vi "GSP_GT_Global.vi"() -> ()   [LabVIEW 2015]
uses:
  SystemUtil/MotorStates.ctl
  SystemUtil/ThreadStates.ctl
panel:
  in  "Grating #":i32
  in  "Grating Name":string
  in  "GT Thread state":T1
  in  "Current Grating":T2
  in  "Detent Pos":i32=6580
  in  "GT Motor State":T3
  in  "GT Position":i32
  in  "GT Target":i32
  in  "GT CPU Temp":dbl
  out "GT Online":bool
  in  "Grating#":i32
  in  "Offset to Clear Pos":i32=6580
  in  "Offset between positions":i32=48715
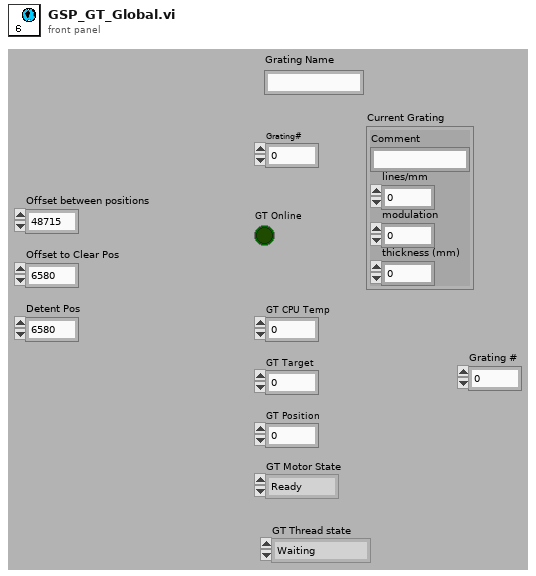
[diagram p1: front panel]
types:
  T1 = typedef "ThreadStates.ctl" = enum16{"Waiting", "Scripting", "Uninitialized", "Error"}
  T2 = cluster{"Comment":string, "lines/mm":i32, "modulation":dbl, "thickness (mm)":dbl}
  T3 = typedef "MotorStates.ctl" = enum16{"Ready", "Moving", "Uninitialized", "Error"}
diagram:
